vi "Convert Assert Event Data to Test Case.vi"(7 "Start Time":timestamp, 10 "Assert Event Data":T1={"name"="", "passed"=FALSE, "call-chain"=[], "test-error"={"status"=FALSE, "code"=0, "source"=""}, "timestamp"=timestamp(0 s since 1904-01-01), "assert-id"="", "test-id"="", "time"=-1.0, "message"="", "properties"=variant, "measurements"=variant, "user-defined"=variant}) -> (2 "Test Case":refnum<class "Test Case.lvclass">)   [LabVIEW 2013, in "JUnit Conversion.lvlib"]
uses:
  JUnit Conversion.lvlib
  <vilib>/addons/_JKI Toolkits/Caraya/classes/Test Result/Assert Event Data (Extended).ctl
  JUnit XML/Test Case/Test Case.lvclass
  JUnit XML/Test Case/Test Result.ctl
  <vilib>/addons/_JKI Toolkits/Caraya/classes/Test Result/Test Result.lvclass
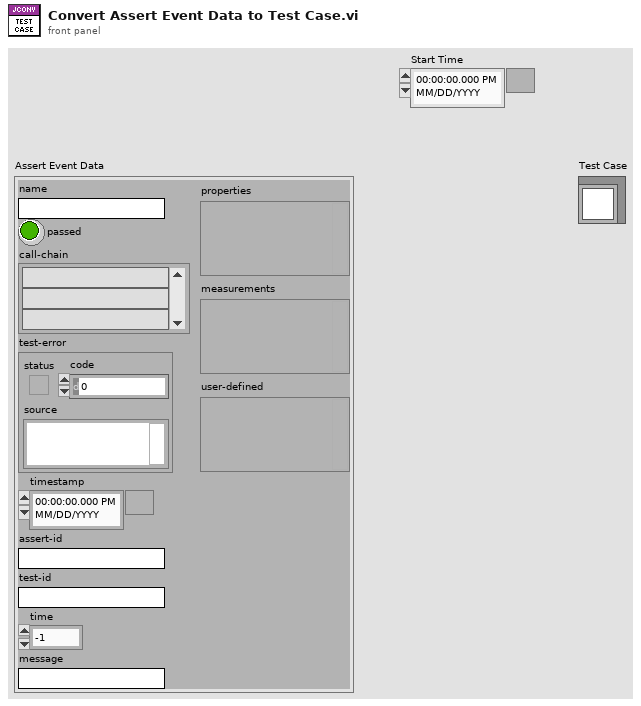
[diagram p1: front panel]
types:
  T1 = typedef "Caraya.lvlib/Test Result.lvclass/Assert Event Data (Extended).ctl" = cluster{"name":string, "passed":bool, "call-chain":string[], "test-error":errorcluster, "timestamp":timestamp, "assert-id":string, "test-id":string, "time":dbl, "message":string, "properties":variant, "measurements":variant, "user-defined":variant}
  T2 = typedef "JUnit XML.lvlib/Test Case.lvclass/Test Result.ctl" = enum16{"Success", "Failure", "Error", "Skipped"}
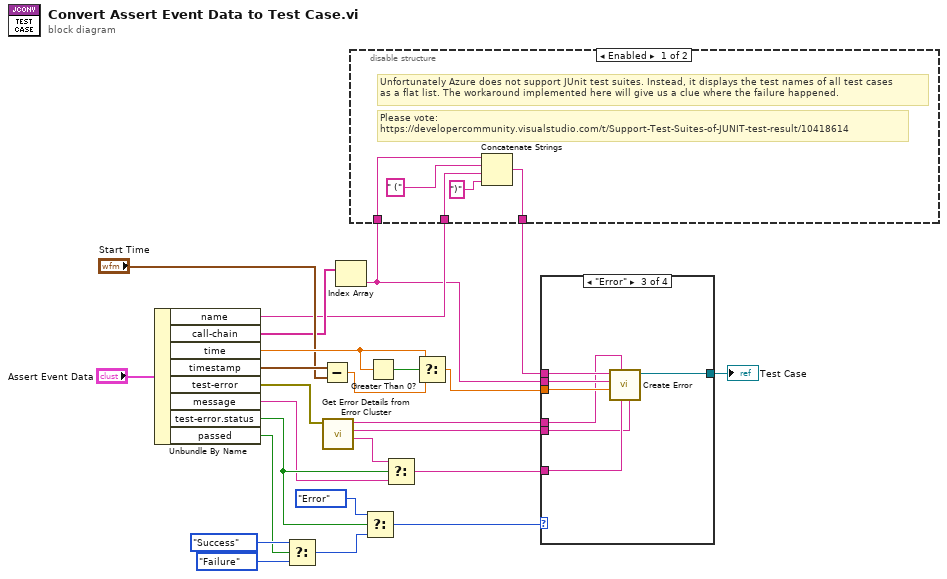
[diagram p0: block diagram]
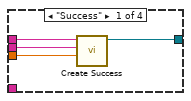
[diagram p2: hidden frame]
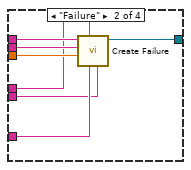
[diagram p3: hidden frame]
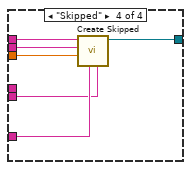
[diagram p4: hidden frame]
diagram:
  n1 = Unbundle By Name("Assert Event Data") -> ("name"=w9:string, "call-chain"=w10:string[], "time"=w18:dbl, "timestamp"=w13:timestamp, "test-error"=w14:errorcluster, "message"=w16:string, "test-error.status"=w17:bool, "passed"=w20:bool)
  n2 = Select(t=Test_Result."Success" ("Test Result"), s=w20, f=Test_Result."Failure" ("Test Result")) -> (s? t:f=w23:T2)
  n3 = Subtract(x=w13, y="Start Time") -> (x-y=w12:dbl)
  n4 = call "Get Error Details from Error Cluster.vi"("error"=w14) -> ("Message"=w15:string, "Call Chain"=w2:string, "Source"=w4:string)  [unwired: 8 in]
  n5 = Index Array(array=w10) -> (element=w1:string)  [unwired: 1 in]
  n6 = disable-structure shown="Enabled" {
    disable-tunnel: w9 -> [w30 w31]
    disable-tunnel: [w28 w31] -> w6
    disable-tunnel: w1 -> [w29 _]
    frame Enabled {
      # "Unfortunately Azure does not support JUnit test suites. Instead, it displays the test names of all test cases\nas a flat list. The workaround implemented here will give us a clue where the failure happened."
      # "Please vote:\nhttps://developercommunity.visualstudio.com/t/Support-Test-Suites-of-JUNIT-test-result/10418614"
      n7 = Concatenate Strings(w29, " (" ("string"), w30, ")" ("string")) -> (w28:string)
    }
    frame Disabled {
    }
  }
  n8 = Select(t=Test_Result."Error" ("Test Result"), s=w17, f=w23) -> (s? t:f=w8:T2)
  n9 = Greater Than 0?(x=w18) -> (x > 0?=w19:bool)
  n10 = Select(t=w15, s=w17, f=w16) -> (s? t:f=w3:string)
  n11 = Select(t=w18, s=w19, f=w12) -> (s? t:f=w5:dbl)
  n12 = case shown="\"Error\"" w8 {
    tunnel: [w35 w42 w49 w55] -> w7
    tunnel: w6 -> [w34 w41 w48 w54]
    tunnel: w1 -> [w33 w40 w47 w53]
    tunnel: w5 -> [w32 w39 w46 w52]
    tunnel: w4 -> [_ w38 w45 _]
    tunnel: w3 -> [_ w37 w44 w51]
    tunnel: w2 -> [_ w36 w43 w50]
    frame "Success" {
      n13 = call "Create Success.vi"("Time"=w32, "Classname"=w33, "Name"=w34) -> ("Test Case"=w35:refnum<class "Test Case.lvclass">)  [unwired: 7 in, 1 out]
    }
    frame "Failure" {
      n14 = call "Create Failure.vi"("Stack Trace"=w36, "Message"=w37, "Type"=w38, "Time"=w39, "Classname"=w40, "Name"=w41) -> ("Test Case"=w42:refnum<class "Test Case.lvclass">)  [unwired: 4 in, 1 out]
    }
    frame "Error" {
      n15 = call "Create Error.vi"("Stack Trace"=w43, "Message"=w44, "Type"=w45, "Time"=w46, "Classname"=w47, "Name"=w48) -> ("Test Case"=w49:refnum<class "Test Case.lvclass">)  [unwired: 4 in, 1 out]
    }
    frame "Skipped" {
      n16 = call "Create Skipped.vi"("Stack Trace"=w50, "Message"=w51, "Time"=w52, "Classname"=w53, "Name"=w54) -> ("Test Case"=w55:refnum<class "Test Case.lvclass">)  [unwired: 5 in, 1 out]
    }
  }
  "Test Case" <- w7
